vi "run.vi"(8 "error in (no error)":errorcluster caption="错误输入（无错误）", 11 "生命游戏 输入":refnum<class "生命游戏.lvclass">) -> (0 "error out":errorcluster caption="错误输出", 3 "生命游戏 输出":refnum<class "生命游戏.lvclass">)   [LabVIEW 2015, in "生命游戏.lvlib" / "生命游戏.lvclass"]
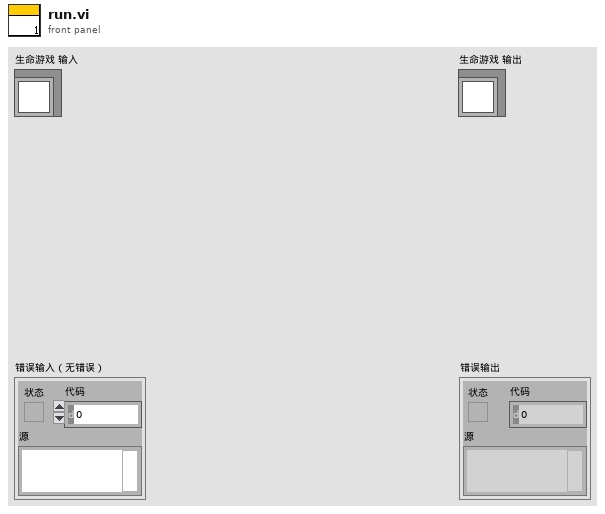
[diagram p1: front panel]
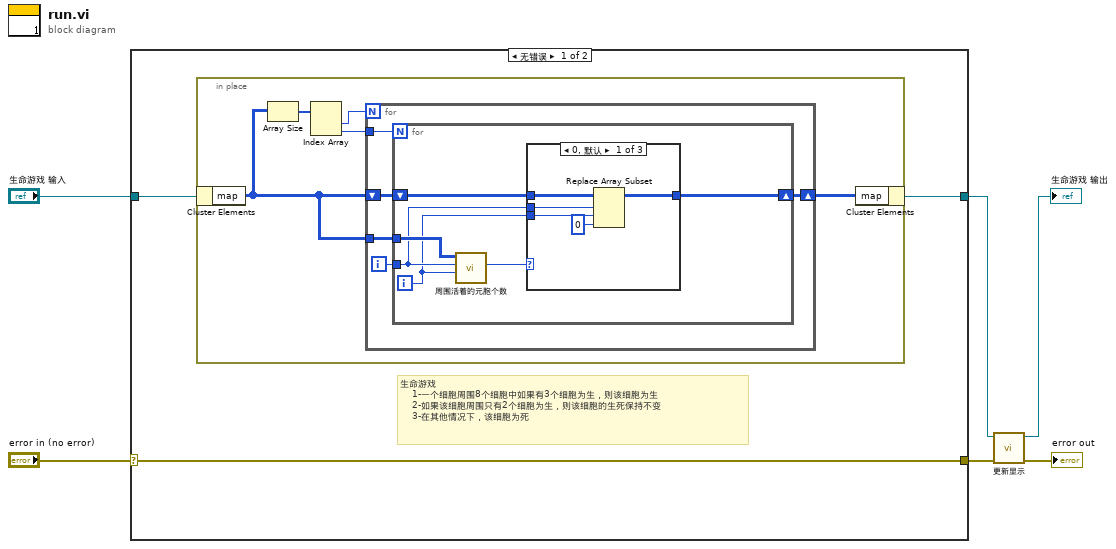
[diagram p0: block diagram]
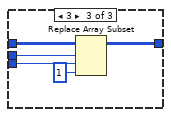
[diagram p3: hidden frame]
diagram:
  n1 = case shown="无错误" "error in (no error)" {
    selector: "error in (no error)" -> [w9 w38]
    tunnel: [w9 w38] -> w4
    tunnel: [w7 w37] -> w2
    tunnel: "生命游戏 输入" -> [w8 w37]
    frame No Error {
      # "生命游戏 \n    1-一个细胞周围8个细胞中如果有3个细胞为生，则该细胞为生\n    2-如果该细胞周围只有2个细胞为生，则该细胞的生死保持不变\n    3-在其他情况下，该细胞为死"
      n2 = in-place {
        n3 = in-place-cluster #1(w8) -> ("map"=w10:u8[][])
        n4 = Array Size(array=w10) -> (size(s)=w14:i32[])
        n5 = Index Array(array=w14) -> (element #1=w13:i32, element #2=w12:i32)  [unwired: 2 in]
        n6 = for {
          N: w13 -> [_]
          tunnel: w12 -> [w19]
          shift-right: [w16] -> w11
          shift-left: w10 -> [w17]
          tunnel: w10 -> [w15]
          i -> [w18]
          n7 = for {
            N: w19 -> [_]
            tunnel: w18 -> [w21]
            shift-right: [w22] -> w16
            shift-left: w17 -> [w24]
            tunnel: w15 -> [w23]
            i -> [w20]
            n8 = call "周围活着的元胞个数.vi"("j"=w20, "i"=w21, "map输入"=w23) -> ("num"=w25:u8)  [unwired: 8 in]
            n9 = case shown="0, 默认" w25 {
              tunnel: w24 -> [w30 w31 w36]
              tunnel: [w29 w31 w35] -> w22
              tunnel: w21 -> [w28 _ w34]
              tunnel: w20 -> [w27 _ w33]
              frame 0, Default {
                n10 = Replace Array Subset(array=w30, new element=u8 0 ("新元素/子数组"), index (row)=w28, index (col)=w27) -> (w29:u8[][])
              }
              frame 2 {
              }
              frame 3 {
                n11 = Replace Array Subset(array=w36, new element=u8 1 ("新元素/子数组"), index (row)=w34, index (col)=w33) -> (w35:u8[][])
              }
            }
          }
        }
        n12 = in-place-cluster #1("map"=w11) -> (w7:refnum<class "生命游戏.lvclass">)
      }
    }
    frame Error {
    }
  }
  n13 = call "更新显示.vi"("error in (no error)"=w4, "生命游戏 输入"=w2) -> ("error out"=→"error out":errorcluster, "生命游戏 输出"=→"生命游戏 输出":refnum<class "生命游戏.lvclass">)  [unwired: 8 in]
